vi "3DScanPath.vi"() -> ()   [LabVIEW 2022 SP3]
uses:
  <vilib>/Platform/NI_3dgraph.lvlib
panel:
  in  "number of points":i16=1000
  in  "Radius at start":i16=1
  in  "Time of scan (s)":i16=1
  in  "Revs per second":i16=10
  in  "CW3DGraphLib._DCWGraph3D":refnum<k7>(container)
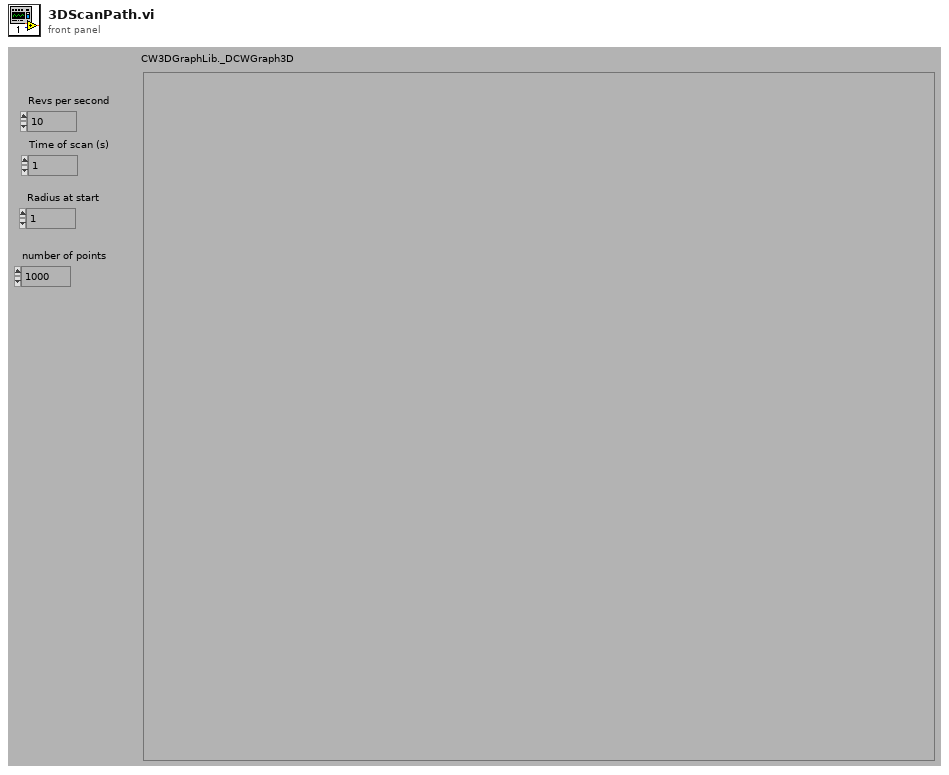
[diagram p1: front panel]
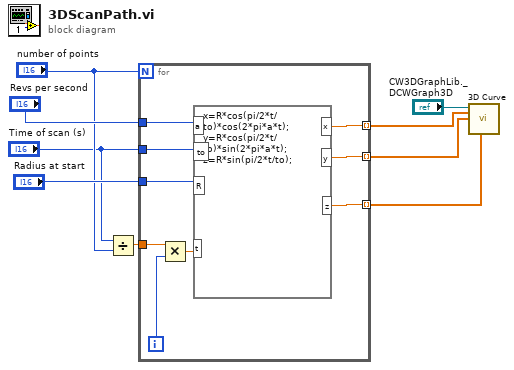
[diagram p0: block diagram]
diagram:
  n1 = Divide(x="Time of scan (s)", y="number of points") -> (x/y=w4:dbl)
  n2 = for {
    N: "number of points" -> [_]
    tunnel: "Radius at start" -> [w18]
    tunnel: "Revs per second" -> [w17]
    tunnel: "Time of scan (s)" -> [w16]
    tunnel: w4 -> [w14]
    tunnel: [w12] -> w3 mode=indexing
    tunnel: [w11] -> w2 mode=indexing
    tunnel: [w10] -> w1 mode=indexing
    i -> [w15]
    n3 = Multiply(x=w14, y=w15) -> (x*y=w13:dbl)
    n4 = formula code="x=R*cos(pi/2*t/to)*cos(2*pi*a*t);\ny=R*cos(pi/2*t/to)*sin(2*pi*a*t);\nz=R*sin(pi/2*t/to);"("a"=w17, "to"=w16, "R"=w18, "t"=w13) -> ("x"=w12:dbl, "y"=w11:dbl, "z"=w10:dbl)
  }
  n5 = call <vilib>:"3D Curve.vi"("z vector"=w1, "y vector"=w2, "x vector"=w3, "3D graph"="CW3DGraphLib._DCWGraph3D") -> ()  [unwired: 1 in, 7 out]
